vi "Base64_Decode.vi"(6 "Error In":errorcluster, 7 "buffer in":string) -> (2 "Error Out":errorcluster, 3 "encoded string":string)   [LabVIEW 2018, in "HttpClient_NET.lvlib"]
doc: "<b> </b> <b> </b>\nHttpClient_NET\nJustin Young - Viviota\nCopyright (c) 2021\nLicense: BSD"
uses:
  HttpClient_NET.lvlib
  <vilib>/httpClient/LabVIEWHTTPClient.lvlib
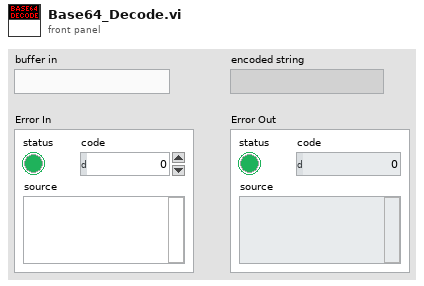
[diagram p1: front panel]
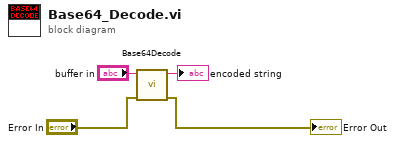
[diagram p0: block diagram]
diagram:
  n1 = call <vilib>:"Base64Decode.vi"("error in (no error)"="Error In", "buffer in"="buffer in") -> ("error out"=→"Error Out":errorcluster, "decoded string"=→"encoded string":string)  [unwired: 8 in]
